vi "Broadcast Response.vi"(8 "error in (no error)":errorcluster, 9 "Acquired Result.lvclass":refnum<class "Acquired Result.lvclass">, 10 "Topic":string, 11 "Channel Scanner in":refnum<class "Channel Scanner.lvclass">) -> (0 "error out":errorcluster, 3 "Channel Scanner out":refnum<class "Channel Scanner.lvclass">)   [LabVIEW 2016, in "Channel Scanner.lvclass"]
uses:
  Channel Scanner.lvclass
  Measure_core/Results/Acquired Result/Acquired Result.lvclass
  Channel Scanner.lvclass/Channel Scanner.ctl
  Read Channel scanner configuration.vi
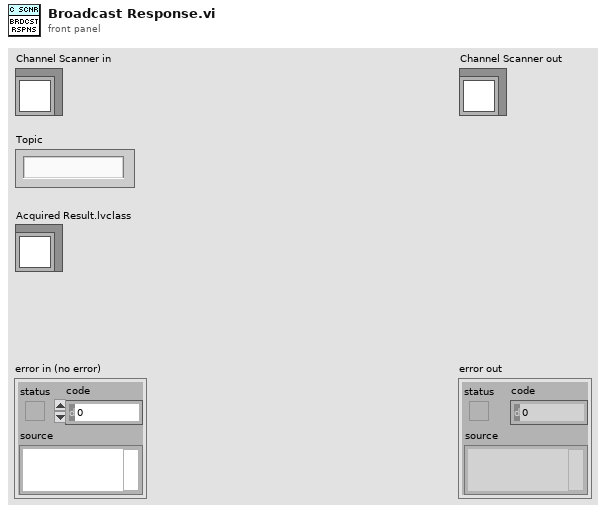
[diagram p1: front panel]
types:
  T1 = typedef "Channel Scanner Configuration.ctl" = cluster{"Scan channels":i32[], "Group with measurement":string}
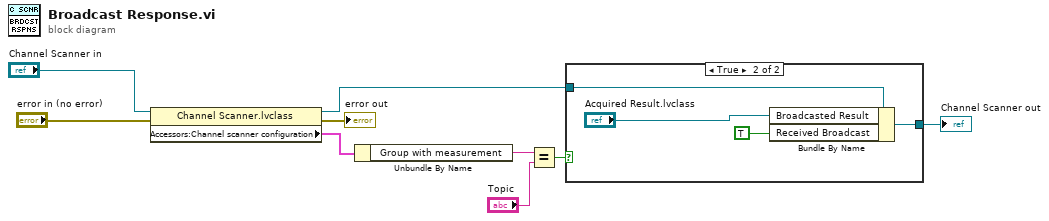
[diagram p0: block diagram]
diagram:
  n1 = property class="Channel Scanner.lvclass"(reference="Channel Scanner in", error in="error in (no error)") -> (reference out=w4:refnum<class "Channel Scanner.lvclass">, error out=→"error out":errorcluster, "Accessors:Channel scanner configuration"=w8:T1)
  n2 = Unbundle By Name(w8) -> ("Group with measurement"=w7:string)
  n3 = Equal?(x=w7, y="Topic") -> (x = y?=w5:bool)
  n4 = case shown="True" w5 {
    tunnel: w4 -> [w10 w14]
    tunnel: [w10 w11] -> w3
    frame False {
    }
    frame True {
      n5 = Bundle By Name(cluster=w14, "Broadcasted Result"="Acquired Result.lvclass", "Received Broadcast"=TRUE) -> (w11:refnum<class "Channel Scanner.lvclass">)
    }
  }
  "Channel Scanner out" <- w3
